vi "Get_YPRHfH.vi"(5 "Device Number":T1, 7 "Update":bool) -> (2 "YRPHfH":T2)   [LabVIEW 2025]
doc: "This navX VI returns the Yaw, Roll, Pitch, Heading, Fused Heading of the navX."
uses:
  _TypeDefs/FRIC_navX_DeviceNumbersTypeDef.ctl
  _TypeDefs/Z900_navX_DeviceRegisters.ctl
  _Util/Z900_navX_Util_LittleEndian_to_BigEndian.vi
  _Internal/FRIC_navX_Get_Registry.vi
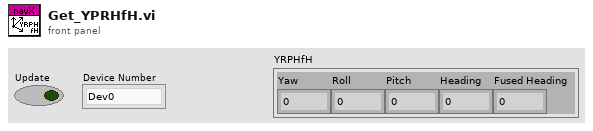
[diagram p1: front panel]
types:
  T1 = typedef "FRIC_navX_DeviceNumbersTypeDef.ctl" = enum16{"Dev0", "Dev1", "Dev2", "Dev3"}
  T2 = cluster{"Yaw":dbl, "Roll":dbl, "Pitch":dbl, "Heading":dbl, "Fused Heading":dbl}
  T3 = typedef "Z900_navX_DeviceRegisters.ctl" = u8
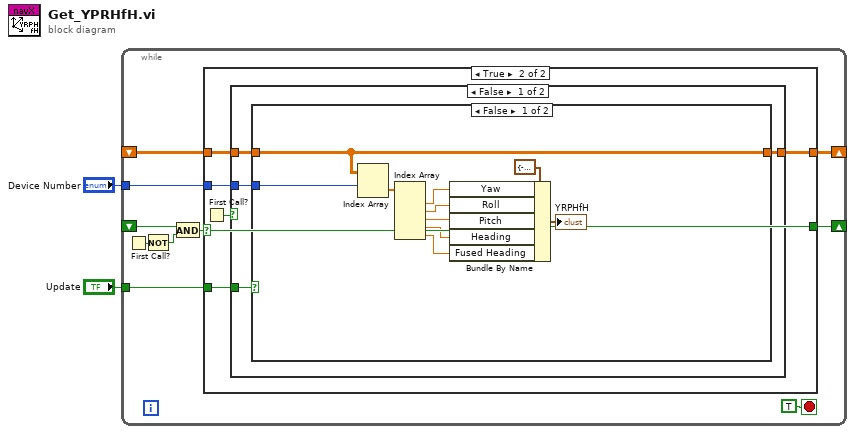
[diagram p0: block diagram]
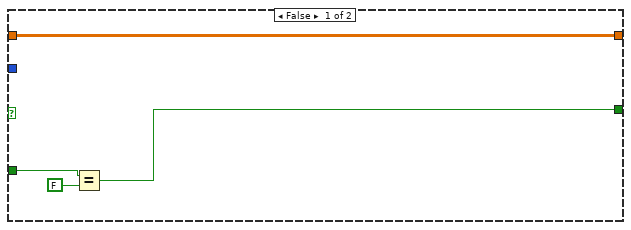
[diagram p2: hidden frame]
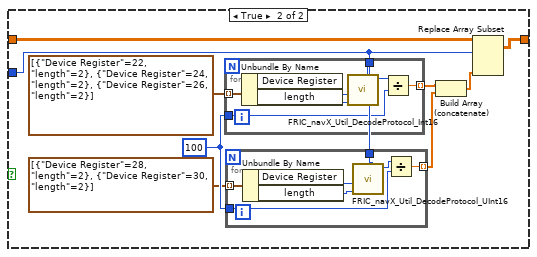
[diagram p3: hidden frame]
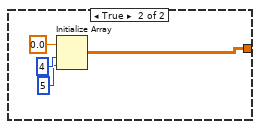
[diagram p4: hidden frame]
diagram:
  n1 = while {
    shift-right: [w10] -> _
    shift-left: _ -> [w11]
    tunnel: "Update" -> [w9]
    tunnel: "Device Number" -> [w8]
    shift-right: [w7] -> _
    shift-left: _ -> [w6]
    stop <- TRUE stop-if-true
    n2 = First Call?() -> (First Call?: T/F=w5:bool)
    n3 = Not(x=w5) -> (.not. x?=w4:bool)
    n4 = And(x=w6, y=w4) -> (x .and. y?=w3:bool)
    n5 = case shown="True" w3 {
      selector: w3 -> [_ w17]
      tunnel: w11 -> [w16 w22]
      tunnel: [w16 w21] -> w10
      tunnel: w9 -> [w15 w20]
      tunnel: w8 -> [_ w19]
      tunnel: [w13 w17] -> w7
      frame False {
        n6 = Equal?(x=w15, y=FALSE) -> (x = y?=w13:bool)
      }
      frame True {
        n7 = First Call?() -> (First Call?: T/F=w18:bool)
        n8 = case shown="False" w18 {
          tunnel: w22 -> [w26 _]
          tunnel: [w25 w63] -> w21
          tunnel: w20 -> [w23 _]
          tunnel: w19 -> [w24 _]
          frame False {
            n9 = case shown="False" w23 {
              tunnel: [w36 w43] -> w25
              tunnel: w26 -> [w36 w45]
              tunnel: w24 -> [w35 w44]
              frame False {
                n10 = Index Array(array=w36, index (row)=w35) -> (element=w32:dbl[])  [unwired: 1 in]
                n11 = Index Array(array=w32) -> (element #1=w31:dbl, element #2=w30:dbl, element #3=w29:dbl, element #4=w28:dbl, element #5=w27:dbl)  [unwired: 5 in]
                n12 = Bundle By Name(cluster=T2 {"Yaw"=-0.34, "Roll"=0.2, "Pitch"=0.2, "Heading"=0.0, "Fused Heading"=359.65} ("YRPHfH"), "Yaw"=w31, "Roll"=w30, "Pitch"=w29, "Heading"=w28, "Fused Heading"=w27) -> (→"YRPHfH":T2)
              }
              frame True {
                w41 = 100 ("y")
                n13 = for {
                  tunnel: w44 -> [w51]
                  tunnel: cluster{"Device Register":T3, "length":i32}[] [{"Device Register"=22, "length"=2}, {"Device Register"=24, "length"=2}, {"Device Register"=26, "length"=2}] ("Array") -> [w50] mode=indexing
                  tunnel: w41 -> [w47]
                  tunnel: [w46] -> w39 mode=indexing
                  n14 = Unbundle By Name(w50) -> ("Device Register"=w49:T3, "length"=w52:i32)
                  n15 = call "FRIC_navX_Util_DecodeProtocol_Int16.vi"("Device Number"=w51, "length"=w52, "Device Register"=w49) -> ("Value"=w48:i16)  [unwired: 8 in]
                  n16 = Divide(x=w48, y=w47) -> (x/y=w46:dbl)
                }
                n17 = for {
                  tunnel: cluster{"Device Register":T3, "length":i32}[] [{"Device Register"=28, "length"=2}, {"Device Register"=30, "length"=2}] ("Array") -> [w59] mode=indexing
                  tunnel: w44 -> [w56]
                  tunnel: w41 -> [w54]
                  tunnel: [w53] -> w38 mode=indexing
                  n18 = Unbundle By Name(w59) -> ("Device Register"=w58:T3, "length"=w57:i32)
                  n19 = call "FRIC_navX_Util_DecodeProtocol_UInt16.vi"("Device Number"=w56, "length"=w57, "Device Register"=w58) -> ("Value"=w55:u16)  [unwired: 8 in]
                  n20 = Divide(x=w55, y=w54) -> (x/y=w53:dbl)
                }
                n21 = Build Array (concatenate)(w39, w38) -> (w37:dbl[])
                n22 = Replace Array Subset(array=w45, new element=w37, index (row)=w44) -> (w43:dbl[][])  [unwired: 1 in]
              }
            }
          }
          frame True {
            n23 = Initialize Array(0.0, 4, 5 ("dimension size")) -> (w63:dbl[][])
          }
        }
      }
    }
  }
